vi "Alignment Mode Window.vi"() -> ()   [LabVIEW 2018]
uses:
  Type Defs/Calibration Values.ctl
panel:
  in  "Cancel Button":bool
  out "CHART":T1(graph) caption="Waveform Chart - dark"
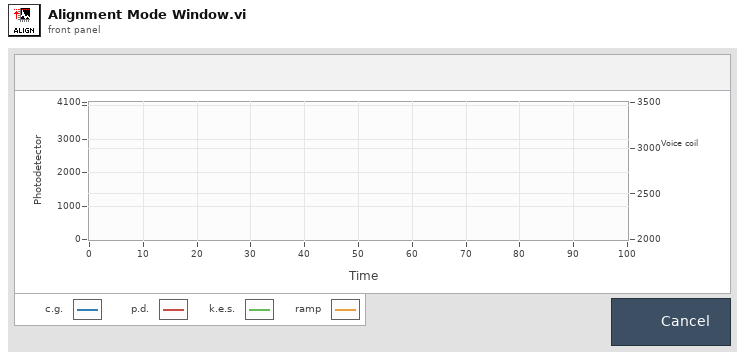
[diagram p1: front panel]
types:
  T1 = cluster{"cap probe":i16, "photodetector":i16, "knife edge sensor":i16, "Ramp Voltage":u16}
  T2 = typedef "Calibration Values.ctl" = cluster{"cap probe":i16, "photodetector":i16, "knife edge sensor":i16, "Ramp Voltage":u16}
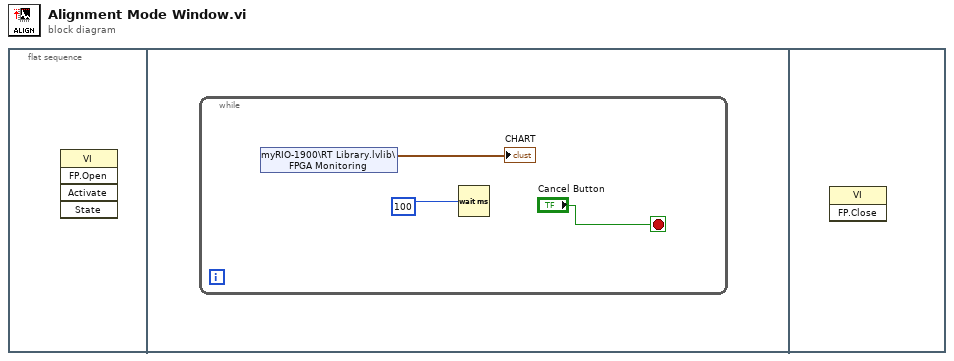
[diagram p0: block diagram]
diagram:
  n1 = flat-sequence {
    frame #0 {
      n2 = invoke class="VI" method="FP.Open"() -> ()  [unwired: 5 in, 5 out]
    }
    frame #1 {
      n3 = while {
        stop <- "Cancel Button" stop-if-true
        n4 = shared-variable "myRIO-1900\\RT Library.lvlib\\FPGA Monitoring"() -> (→"CHART":T2)  [unwired: 1 in, 1 out]
        n5 = Wait (ms)(milliseconds to wait=100) -> ()  [unwired: 1 out]
      }
    }
    frame #2 {
      n6 = invoke class="VI" method="FP.Close"() -> ()  [unwired: 3 in, 3 out]
    }
  }
